vi "Dock Child.vi"(0 "LV MDI in":refnum<class "LV MDI.lvclass">, 5 "Child Hwnd":u32, 7 "Dock?":bool, 11 "error in (no error)":errorcluster) -> (4 "LV MDI out":refnum<class "LV MDI.lvclass">, 15 "error out":errorcluster)   [LabVIEW 2016, in "LV MDI.lvclass"]
doc: "Dock?Undock chilsd window."
uses:
  LV MDI.lvclass
  LV MDI.lvclass/LV MDI.ctl
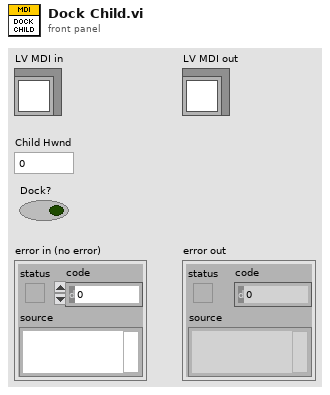
[diagram p1: front panel]
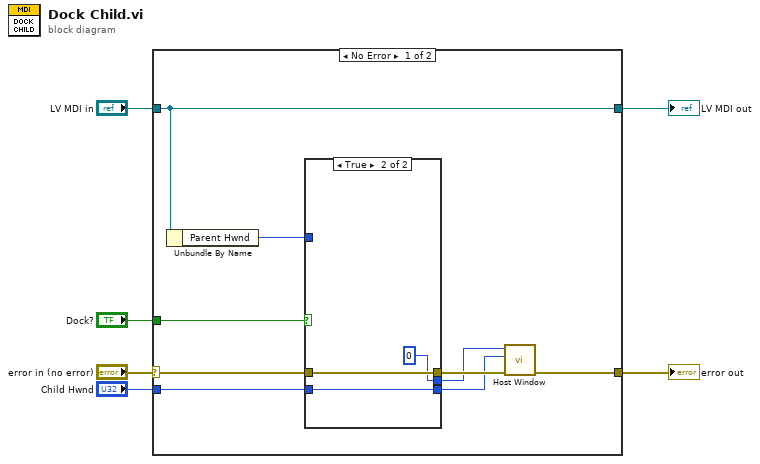
[diagram p0: block diagram]
diagram:
  n1 = case shown="No Error" "error in (no error)" {
    selector: "error in (no error)" -> [w11 w23]
    tunnel: [w10 w23] -> w5
    tunnel: [w15 w22] -> w3
    tunnel: "LV MDI in" -> [w15 w22]
    tunnel: "Child Hwnd" -> [w12 _]
    tunnel: "Dock?" -> [w13 _]
    frame No Error {
      n2 = Unbundle By Name(w15) -> ("Parent Hwnd"=w14:i32)
      n3 = case shown="True" w13 {
        tunnel: w11 -> [w18 w21]
        tunnel: [w18 w21] -> w9
        tunnel: [w17 w20] -> w8
        tunnel: [w16 0 ("hWnd")] -> w7
        tunnel: w12 -> [w17 w20]
        tunnel: w14 -> [w16 _]
        frame False {
        }
        frame True {
        }
      }
      n4 = call "Host Window.vi"("error in (no error)"=w9, "Child Hwnd"=w8, "Parent Hwnd"=w7) -> ("error out"=w10:errorcluster)  [unwired: 8 in]
    }
    frame Error {
    }
  }
  "error out" <- w5
  "LV MDI out" <- w3
